vi "1_While loop & charts(170382,170307).vi"() -> ()   [LabVIEW 2015]
panel:
  in  "stop":bool
  out "Sweep chart":dbl(graph)=3.1699444888479555
  out "Scope chart":dbl(graph)=3.1699444888479555
  out "Strip chart":dbl(graph)=3.1699444888479555
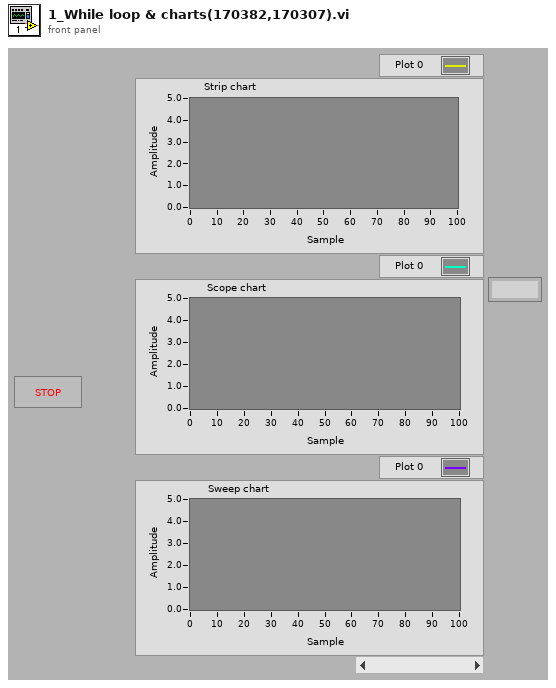
[diagram p1: front panel]
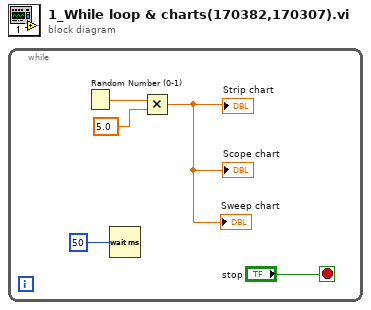
[diagram p0: block diagram]
diagram:
  n1 = while {
    stop <- "stop" stop-if-true
    n2 = Random Number (0-1)() -> (number: 0 to 1=w5:dbl)
    n3 = Wait (ms)(milliseconds to wait=u32 50) -> ()  [unwired: 1 out]
    n4 = Multiply(x=w5, y=5.0) -> (x*y=→"Strip chart" →"Scope chart" →"Sweep chart":dbl)
  }
